vi "Event Handler.vi"(8 "error in (no error)":errorcluster, 10 "Stop Event Handler":refnum<user-event>, 11 "ScrollZoomGraphChart in":refnum<class "ScrollZoomGraphChart.lvclass">=refnum) -> (0 "error out":errorcluster)   [LabVIEW 2023, in "ScrollZoomGraphChart.lvclass"]
doc: "The <b>Event Handler VI</b> is a dynamic dispatch VI that should be overwritten if events are needed to create the enhanced QControl. \n\nBy inheriting from the main Control.lvclass the overwritten <b>Event Handler VI</b> will be launched asynchronously in the initialization of the QControl.\n<b> </b> <b> </b>\n©2016 Q Software Innovations, LLC (QSI)\nwritten by Quentin Alldredge\nproduced in LabVIEW 2015\n\nsupport@qsoftwareinnovations.com\nwww.qsoftwareinnovations.com\n\nAll rights reserved.\n\nRedistribution and use in source and binary forms, with or without modification, are permitted provided that the following conditions are met:\n\n * Redistributions of source code must retain the above copyright notice, this list of conditions and the following disclaimer.\n * Redistributions in binary form must reproduce the above copyright notice, this list of conditions and the following disclaimer in the documentation and/or other materials provided with the distribution.\n * Neither the name of Q Software Innovations, LLC. nor the names of its contributors may be used to endorse or promote products derived from this software without specific prior written permission.\n\nTHIS SOFTWARE IS PROVIDED BY THE COPYRIGHT HOLDERS AND CONTRIBUTORS \"AS IS\" AND ANY EXPRESS OR IMPLIED WARRANTIES, INCLUDING, BUT NOT LIMITED TO, THE IMPLIED WARRANTIES OF MERCHANTABILITY AND FITNESS FOR A PARTICULAR PURPOSE ARE DISCLAIMED. IN NO EVENT SHALL THE COPYRIGHT OWNER OR CONTRIBUTORS BE LIABLE FOR ANY DIRECT, INDIRECT, INCIDENTAL, SPECIAL, EXEMPLARY, OR CONSEQUENTIAL DAMAGES (INCLUDING, BUT NOT LIMITED TO, PROCUREMENT OF SUBSTITUTE GOODS OR SERVICES; LOSS OF USE, DATA, OR PROFITS; OR BUSINESS INTERRUPTION) HOWEVER CAUSED AND ON ANY THEORY OF LIABILITY, WHETHER IN CONTRACT, STRICT LIABILITY, OR TORT (INCLUDING NEGLIGENCE OR OTHERWISE) ARISING IN ANY WAY OUT OF THE USE OF THIS SOFTWARE, EVEN IF ADVISED OF THE POSSIBILITY OF SUCH DAMAGE."
uses:
  ScrollZoomGraphChart.lvclass
  <vilib>/Analysis/geometry.llb/Point in Polygon Position.ctl
  <vilib>/Analysis/NI_AAL_Geometry.lvlib
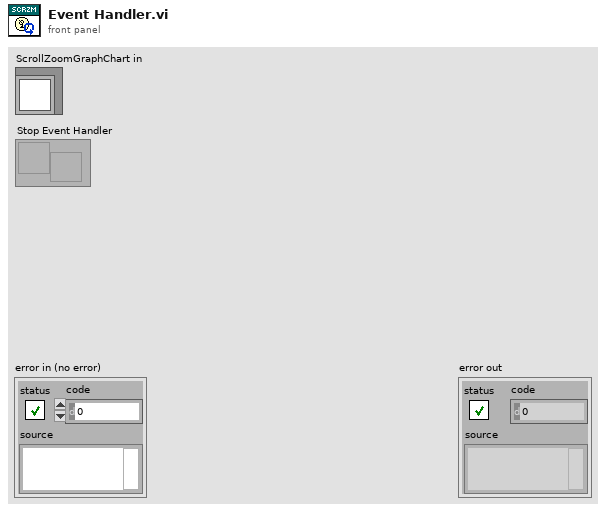
[diagram p1: front panel]
types:
  T1 = typedef "NI_AAL_Geometry.lvlib/Point in Polygon Position.ctl" = u16
  T2 = typedef "LVPoint32TypeDef.ctl" = cluster{"Horizontal":i32, "Vertical":i32}
  T3 = typedef "LVRectTypeDef.ctl" = cluster{"Left":i16, "Top":i16, "Right":i16, "Bottom":i16}
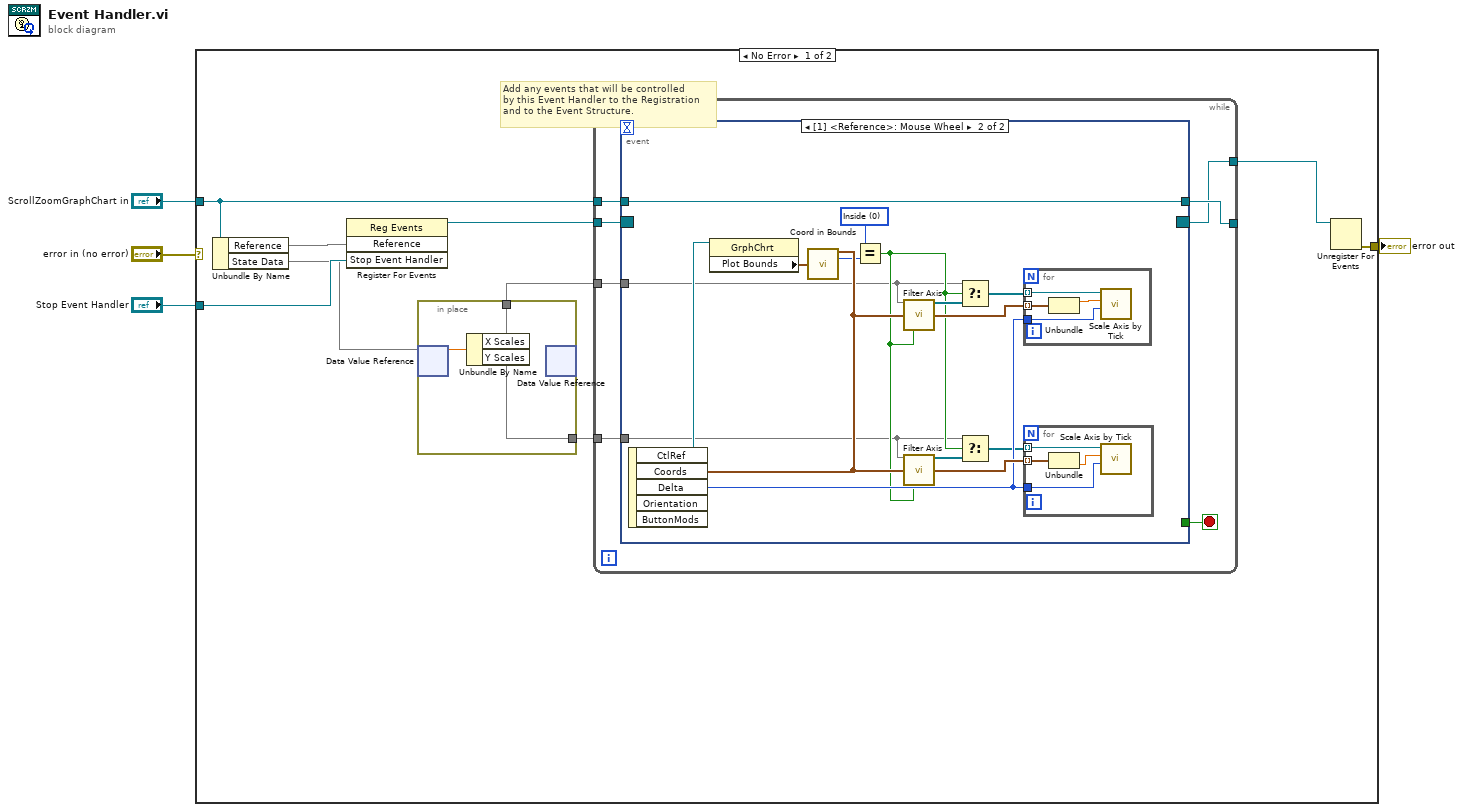
[diagram p0: block diagram]
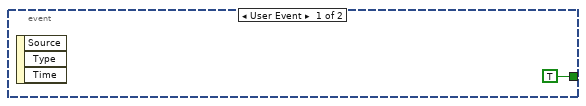
[diagram p2: hidden frame]
diagram:
  n1 = case shown="No Error" "error in (no error)" {
    selector: "error in (no error)" -> [_ w49]
    tunnel: [w13 w49] -> w3
    tunnel: "ScrollZoomGraphChart in" -> [w5 _]
    tunnel: "Stop Event Handler" -> [w11 _]
    frame No Error {
      # "Add any events that will be controlled\nby this Event Handler to the Registration\nand to the Event Structure."
      n2 = Unbundle By Name(w5) -> ("Reference"=w12, "State Data"=w9)
      n3 = register-events(w12, w11) -> (reference out=w10:refnum<event-registration>)  [unwired: 2 in, 1 out]
      n4 = in-place {
        in-place-border: [w15] -> w8
        in-place-border: [w14] -> w7
        n5 = in-place-dvr #1(w9) -> (w16:dbl)  [unwired: 1 out]
        n6 = Unbundle By Name(w16) -> ("X Scales"=w15, "Y Scales"=w14)
        n7 = in-place-dvr #1() -> ()  [unwired: 1 in, 2 out]
      }
      n8 = while {
        tunnel: w8 -> [w22]
        tunnel: w7 -> [w21]
        tunnel: w10 -> [w20]
        tunnel: [w19] -> _
        tunnel: w5 -> [w18]
        tunnel: [w17] -> w6
        stop <- w23 stop-if-true
        n9 = event shown="[1] <Reference>: Mouse Wheel" {
          selector: w20 -> [_ _]
          dyn-events: [_ _] -> w17
          timeout: _ -> [_ _]
          tunnel: [TRUE _] -> w23
          tunnel: w22 -> [_ w27]
          tunnel: w21 -> [_ w26]
          tunnel: [_ w25] -> w19
          tunnel: w18 -> [_ w25]
          event User Event {
            n10 = event-data() -> ()  [unwired: 1 in, 3 out]
          }
          event Mouse Wheel {
            w35 = T1 0 items=["Inside", "On Boundary", "Outside"] ("x")
            n11 = event-data() -> ("CtlRef"=w34:refnum<vi>, "Coords"=w37:T2, "Delta"=w31:i32)  [unwired: 1 in, 2 out]
            n12 = property class="GrphChrt"(reference=w34) -> ("Plot Bounds"=w38:T3)  [unwired: 1 in, 2 out]
            n13 = call "Coord in Bounds.vi"("Coords"=w37, "Plot Bounds"=w38) -> ("position"=w36:T1)  [unwired: 12 in, 1 out]
            n14 = Equal?(x=w35, y=w36) -> (x = y?=w28:bool)
            n15 = call "Filter Axis.vi"("Graph Scale in"=w27, "Coords"=w37, "Bypass Filter"=w28) -> ("Filter Graph Scale out"=w40:refnum<vi>[], "Axis Value"=w39:cluster{"X":dbl, "Y":dbl}[])  [unwired: 10 in, 1 out]
            n16 = call "Filter Axis.vi"("Graph Scale in"=w26, "Coords"=w37, "Bypass Filter"=w28) -> ("Filter Graph Scale out"=w33:refnum<vi>[], "Axis Value"=w32:cluster{"X":dbl, "Y":dbl}[])  [unwired: 10 in, 1 out]
            n17 = Select(t=w27, s=w28, f=w40) -> (s? t:f=w30:refnum<vi>[])
            n18 = Select(t=w26, s=w28, f=w33) -> (s? t:f=w29:refnum<vi>[])
            n19 = for {
              tunnel: w30 -> [w48] mode=indexing
              tunnel: w39 -> [w47] mode=indexing
              tunnel: w31 -> [w45]
              n20 = Unbundle(w47) -> ("X"=w46:dbl)  [unwired: 1 out]
              n21 = call "Scale Axis by Tick.vi"("Tick Scale"=w45, "Axis Focus Value"=w46, "GraphScale in"=w48) -> ()  [unwired: 9 in]
            }
            n22 = for {
              tunnel: w29 -> [w44] mode=indexing
              tunnel: w32 -> [w43] mode=indexing
              tunnel: w31 -> [w42]
              n23 = Unbundle(w43) -> ("Y"=w41:dbl)  [unwired: 1 out]
              n24 = call "Scale Axis by Tick.vi"("Tick Scale"=w42, "Axis Focus Value"=w41, "GraphScale in"=w44) -> ()  [unwired: 9 in]
            }
          }
        }
      }
      n25 = Unregister For Events(event registration refnum=w6) -> (error out=w13:errorcluster)  [unwired: 1 in]
    }
    frame Error {
    }
  }
  "error out" <- w3
